vi "SubVi lightshadecontrol.vi"(11 "Control panel":T1) -> (0 "LED 4":cluster{"Color":u32, "Color":u32}[](array[cluster]), 1 "LED 3":cluster{"Color":u32, "Color":u32}[](array[cluster]), 2 "LED 2":cluster{"Color":u32, "Color":u32}[](array[cluster]), 3 "LED 1":cluster{"Color":u32, "Color":u32}[](array[cluster]), 4 "LED 5":cluster{"Color":u32, "Color":u32}[](array[cluster]))   [LabVIEW 2020]
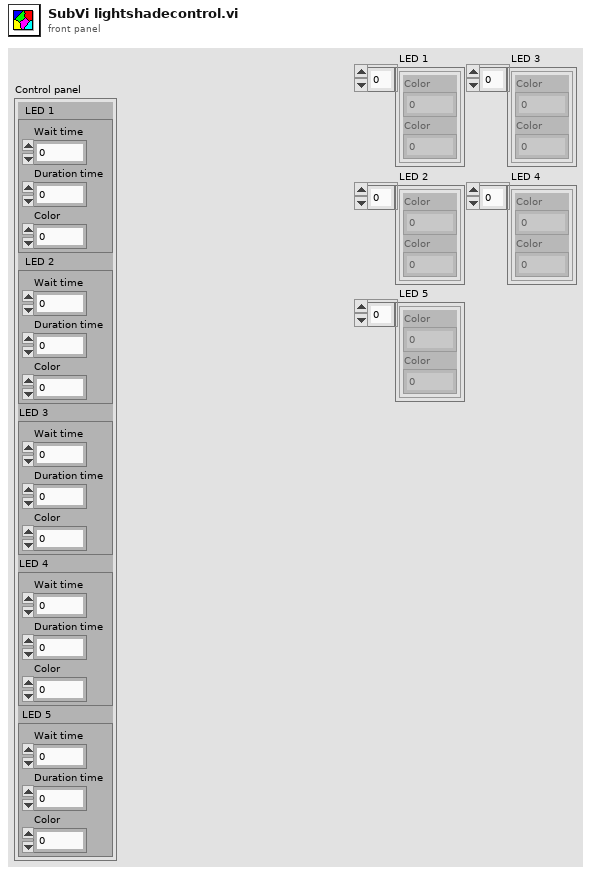
[diagram p1: front panel]
types:
  T1 = cluster{"  LED 1":cluster{"Wait time":dbl, "Duration time":dbl, "Color":u32}, "  LED 2":cluster{"Wait time":dbl, "Duration time":dbl, "Color":u32}, "LED 3":cluster{"Wait time":dbl, "Duration time":dbl, "Color":u32}, "LED 4":cluster{"Wait time":dbl, "Duration time":dbl, "Color":u32}, " LED 5":cluster{"Wait time":dbl, "Duration time":dbl, "Color":u32}}
  T2 = cluster{"Wait time":dbl, "Duration time":dbl, "Color":u32}
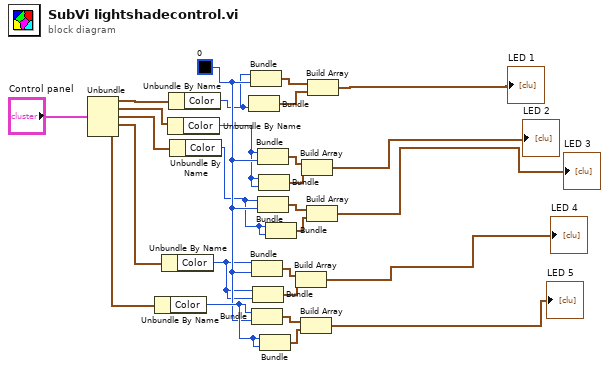
[diagram p0: block diagram]
diagram:
  w25 = u32 0
  n1 = Unbundle("Control panel") -> ("LED 1"=w6:T2, "LED 2"=w10:T2, "LED 3"=w14:T2, "LED 4"=w22:T2, "LED 5"=w23:T2)
  n2 = Unbundle By Name(w23) -> ("Color"=w26:u32)
  n3 = Unbundle By Name(w22) -> ("Color"=w24:u32)
  n4 = Unbundle By Name(w10) -> ("Color"=w13:u32)
  n5 = Unbundle By Name(w6) -> ("Color"=w7:u32)
  n6 = Unbundle By Name(w14) -> ("Color"=w17:u32)
  n7 = Bundle("Color"=w7, "Color"=w7) -> (w9:cluster{"Color":u32, "Color":u32})  [unwired: 1 in]
  n8 = Bundle("Color"=w7, w25) -> (w8:cluster{"Color":u32, u32})  [unwired: 1 in]
  n9 = Bundle("Color"=w24, w25) -> (w18:cluster{"Color":u32, u32})  [unwired: 1 in]
  n10 = Bundle("Color"=w26, w25) -> (w20:cluster{"Color":u32, u32})  [unwired: 1 in]
  n11 = Bundle("Color"=w24, "Color"=w24) -> (w19:cluster{"Color":u32, "Color":u32})  [unwired: 1 in]
  n12 = Bundle("Color"=w13, w25) -> (w11:cluster{"Color":u32, u32})  [unwired: 1 in]
  n13 = Bundle("Color"=w17, w25) -> (w15:cluster{"Color":u32, u32})  [unwired: 1 in]
  n14 = Bundle("Color"=w13, "Color"=w13) -> (w12:cluster{"Color":u32, "Color":u32})  [unwired: 1 in]
  n15 = Bundle("Color"=w26, "Color"=w26) -> (w21:cluster{"Color":u32, "Color":u32})  [unwired: 1 in]
  n16 = Bundle("Color"=w17, "Color"=w17) -> (w16:cluster{"Color":u32, "Color":u32})  [unwired: 1 in]
  n17 = Build Array(w18, w19) -> (→"LED 4":cluster{"Color":u32, "Color":u32}[])
  n18 = Build Array(w20, w21) -> (→"LED 5":cluster{"Color":u32, "Color":u32}[])
  n19 = Build Array(w11, w12) -> (→"LED 2":cluster{"Color":u32, "Color":u32}[])
  n20 = Build Array(w15, w16) -> (→"LED 3":cluster{"Color":u32, "Color":u32}[])
  n21 = Build Array(w8, w9) -> (→"LED 1":cluster{"Color":u32, "Color":u32}[])
